vi "GetDeviceKeys.vi"(4 "error in (no error)":errorcluster, 7 "CmdLib In":refnum<k24>) -> (0 "error out":errorcluster, 1 "Device Keys":string[](array[string]), 3 "CmdLib Out":refnum<k24>)   [LabVIEW 2013]
uses:
  C:/Code/Apps/Utilities/AG-UC2-UC8/AG-UC2-UC8/Install/Samples/LabVIEW/LabVIEW 2013/CmdLibAgilis.dll
  CmdLibAgilis.dll
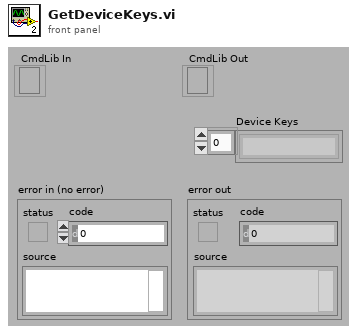
[diagram p1: front panel]
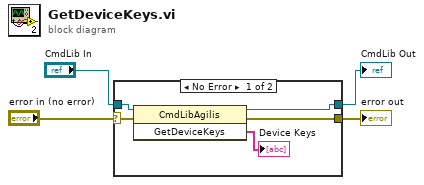
[diagram p0: block diagram]
diagram:
  n1 = case shown="No Error" "error in (no error)" {
    selector: "error in (no error)" -> [w6 w11]
    tunnel: [w5 w11] -> w3
    tunnel: "CmdLib In" -> [w9 w10]
    tunnel: [w8 w10] -> w1
    frame No Error {
      n2 = invoke class="CmdLibAgilis" method="GetDeviceKeys"(reference=w9, error in=w6) -> (reference out=w8:refnum<k24>, error out=w5:errorcluster, "GetDeviceKeys"=→"Device Keys":string[])  [unwired: 1 in]
    }
    frame Error {
    }
  }
  "error out" <- w3
  "CmdLib Out" <- w1
